vi "example.vi"() -> ()   [LabVIEW 2015]
uses:
  SubVI/lstsqr_lines.vi
  SubVI/z-split sum difference.vi
  SubVI/Local gradient preallocation.vi
  <vilib>/vision/NI_Vision_Development_Module.lvlib
panel:
  in  "Image type":u16(ring) items=["Fluorescent", "Brightfield"]
  in  "pattern":string="*.*"
  in  "Current im":u16=5 caption="Current image" max=0 step=1
  out "ImageArray":u16[][][](array[numeric])
  in  "Express btn":bool
  in  "Positive angle":dbl
  out "Show center":bool
  out "Z plot":cluster{i32[], "XYZ":dbl[]}(graph)
  out "Y plot":cluster{i32[], "XYZ":dbl[]}(graph)
  out "X plot":cluster{i32[], "XYZ":dbl[]}(graph)
  out "Gx graph":dbl[][](graph)
  in  "Center size":dbl=5.0 min=1.0 step=2.0
  out "Center":dbl[](array[numeric]) format="%#.5g"
  out "Weights":dbl[](array[numeric])
  out "gradients":dbl[][](array[numeric])
  out "centers":i32[][](array[numeric])
  in  "Gradient btn":bool
  out "Gy graph":dbl[][](graph)
  out "G graph":dbl[][](graph)
  in  "Threshold type":u16(ring) items=["Top fraction", "Top value"]
  in  "Weights type":u16(ring)=1 items=["None", "G", "G^2"]
  in  "Threshold":dbl=2.0
  in  "R":dbl=10.0
  in  "Center Button":bool
  in  "Stop Button":bool
  in  "Read Button":bool
  out "Input image":T1(plugin-control)
  in  "File Path":path
  out "Filtered G":dbl[][](graph)
  # "Run vi. \n1. Use default image or select a greyscale image and click Read. There is an option to select either directory or a file. If directory is selected, Labview will read all the files in the folder AND in ALL subfolders. You can use a \"pattern\" field to select specific files.\n2. Select an image type: Fluorescent or Brightfield (affect z-calculation)\n3. Set parameters R, Threshold, Weights type, Positive angle, etc.\n4. A. Single file\n    OPTION1. Step by step: \n      - click Gradient to calculate local gradient images\n      - click Find center to calculate xyz position of the particle\n    OPTION2. Express: \n      - click Express center\n\n   B. Folder\n    OPTION1. Step by step: \n      - click Gradient to calculate local gradient images for the image selected in Current image\n      - click Find center to calculate xyz position of the particle for the image selected in Current image\n    OPTION2. Express: \n      - click Express center to find center for all the loaded files\n\nAuthor: Anatolii Kashchuk"
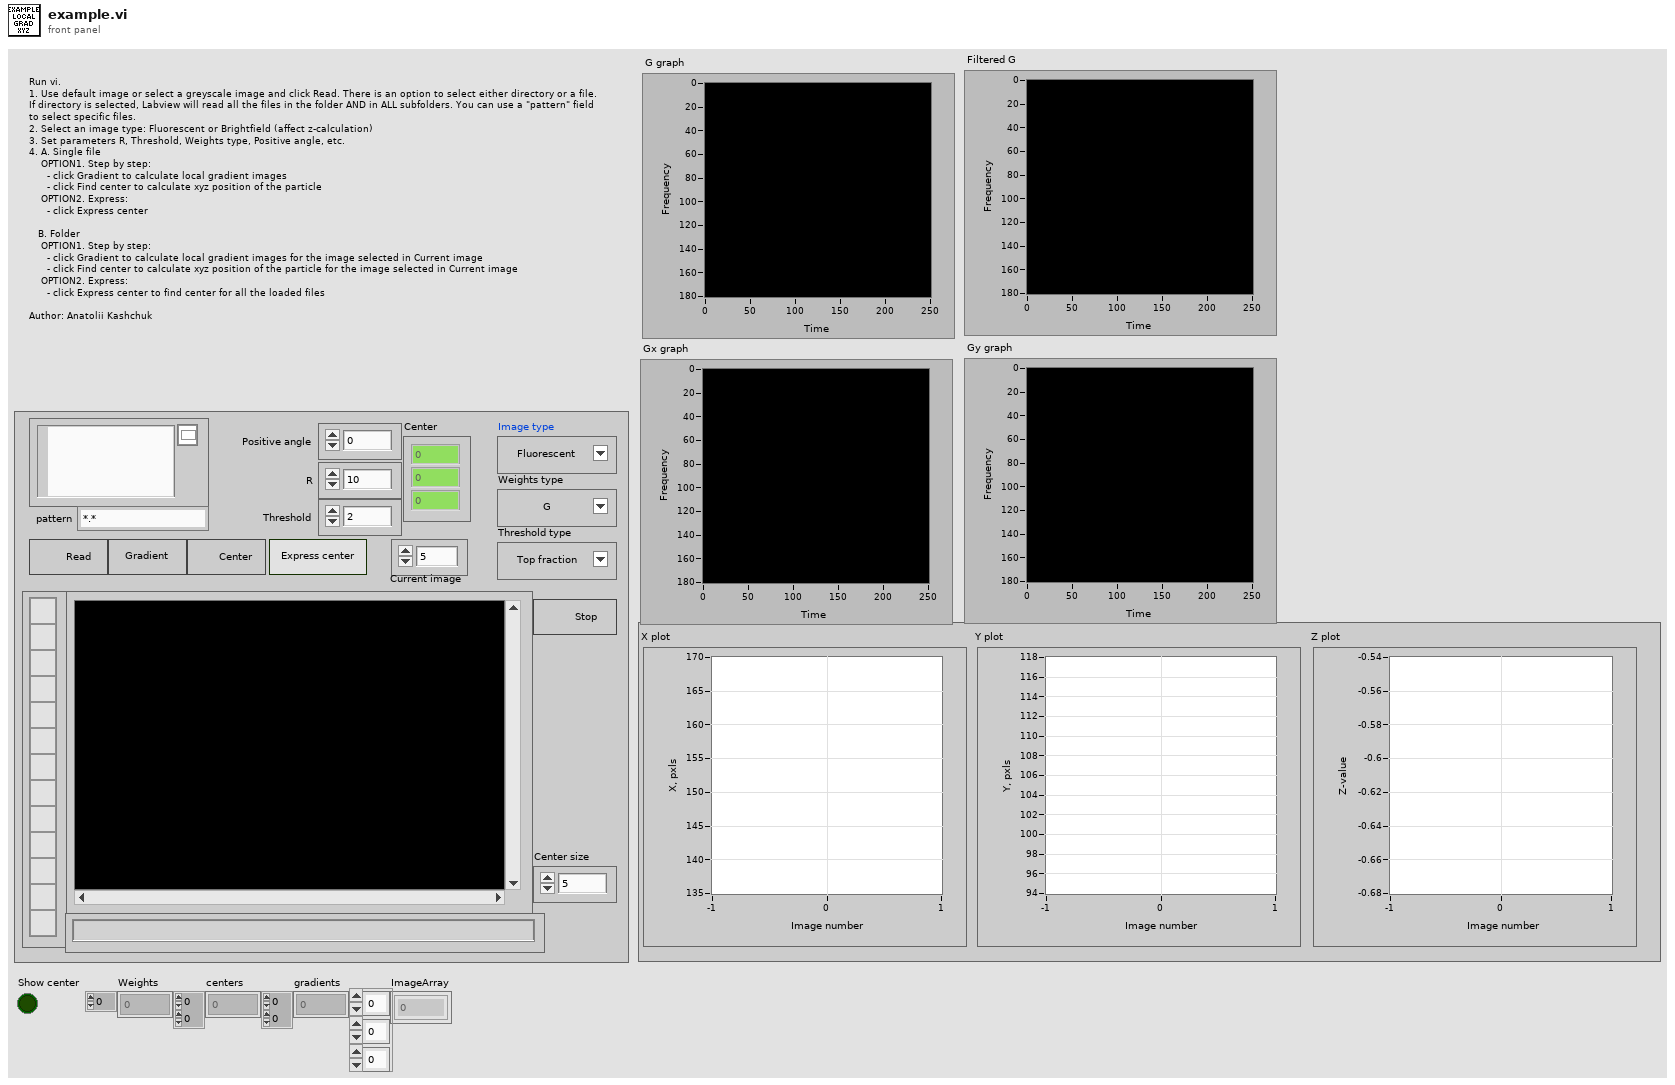
[diagram p1: front panel]
types:
  T1 = typedef "IMAQ Image.ctl" = refnum<image>
  T2 = typedef "Image Type" = u32
  T3 = cluster{"Left":i32, "Top":i32, "Right":i32, "Bottom":i32}
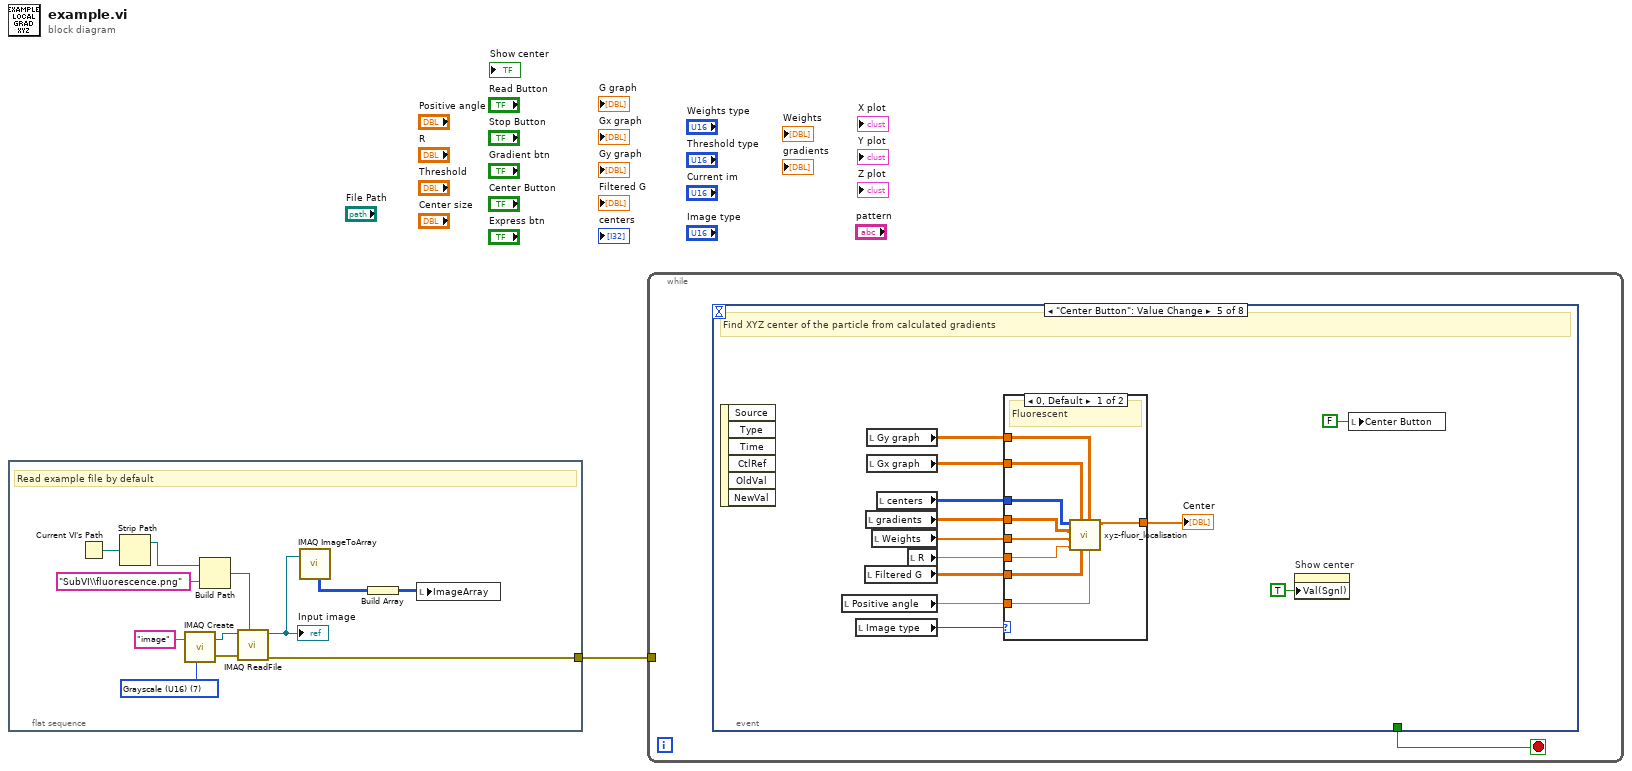
[diagram p0: block diagram]
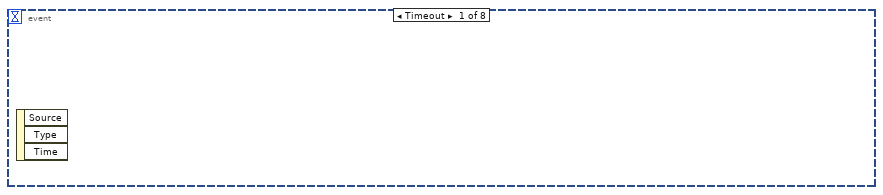
[diagram p2: hidden frame]
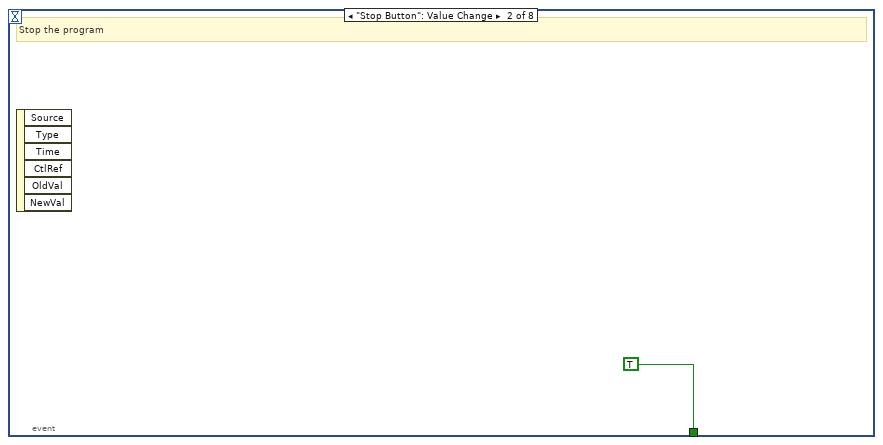
[diagram p3: hidden frame]
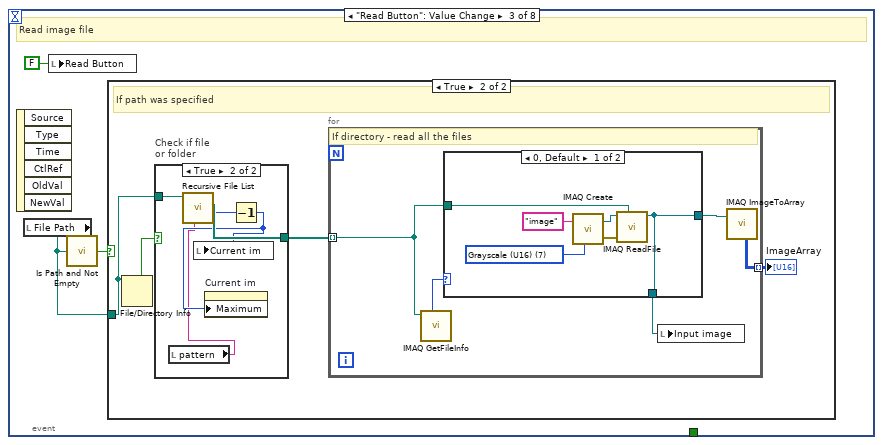
[diagram p4: hidden frame]
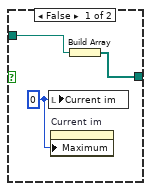
[diagram p6: hidden frame]
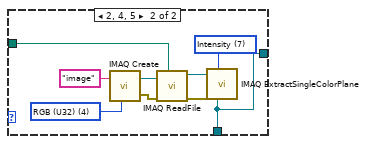
[diagram p7: hidden frame]
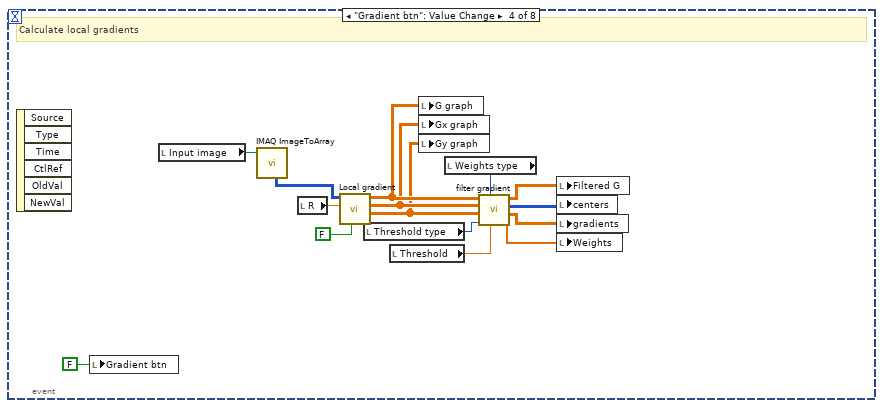
[diagram p8: hidden frame]
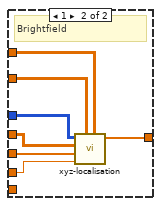
[diagram p9: hidden frame]
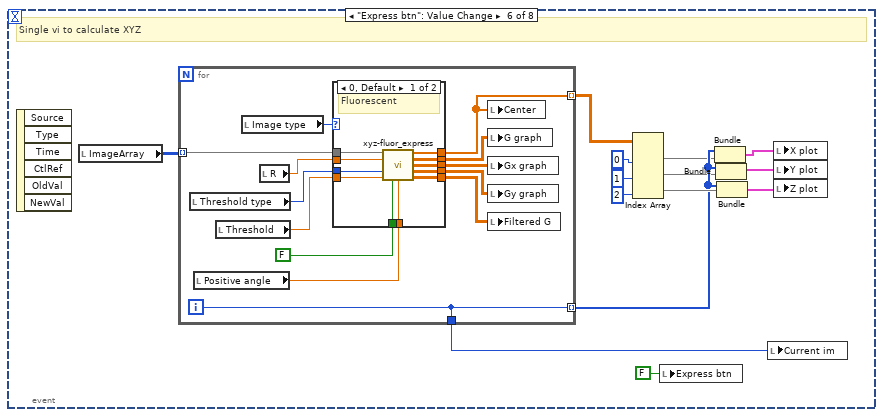
[diagram p10: hidden frame]
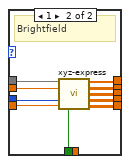
[diagram p11: hidden frame]
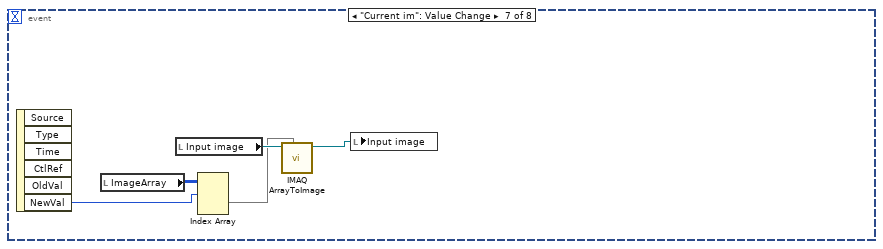
[diagram p12: hidden frame]
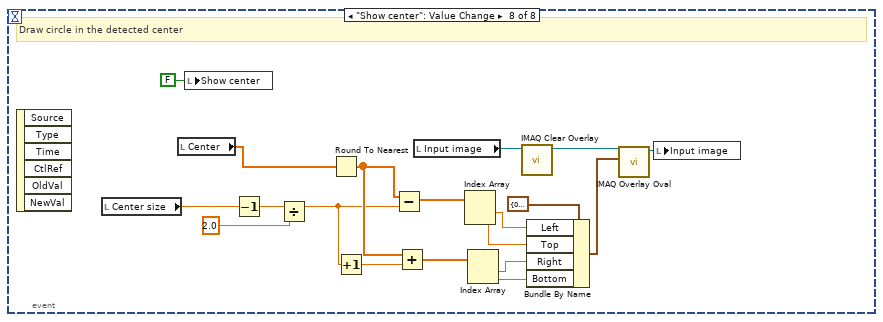
[diagram p13: hidden frame]
diagram:
  n1 = flat-sequence {
    tunnel: [w10] -> w1
    frame #0 {
      w9 = T2 7 items=["Grayscale (U8)", "Grayscale (I16)", "Grayscale (SGL)", "Complex (CSG)", "RGB (U32)", "HSL (U32)", "RGB (U64)", "Grayscale (U16)"] ("Image Type")
      # "Read example file by default"
      n2 = Current VI's Path() -> (path=w7:path)
      n3 = Strip Path(path=w7) -> (stripped path=w5:path)  [unwired: 1 out]
      n4 = call "IMAQ Create"("Image Name"="image", "Image Type"=w9) -> ("New Image"=w11:T1, "error out"=w12:errorcluster)  [unwired: 3 in]
      n5 = Build Path(base path=w5, name or relative path="SubVI\\fluorescence.png") -> (appended path=w6:path)
      n6 = call "IMAQ ReadFile"("File Path"=w6, "error in (no error)"=w12, "Image"=w11) -> ("error out"=w10:errorcluster, "Image Out"=w4:T1)  [unwired: 4 in, 3 out]
      "Input image" <- w4
      n7 = call "IMAQ ImageToArray"("Image"=w4) -> ("Image Pixels (U16)"=w2:u16[][])  [unwired: 3 in, 4 out]
      n8 = Build Array(w2) -> (w3:u16[][][])
      n9 = local write "ImageArray"(w3) -> ()
    }
  }
  n10 = while {
    tunnel: w1 -> [_]
    stop <- w14 stop-if-true
    n11 = event shown="[4] \"Center Button\": Value Change" {
      selector: _ -> [_ _ _ _ _ _ _ _]
      dyn-events: _ -> [_ _ _ _ _ _ _ _]
      timeout: _ -> [_ _ _ _ _ _ _ _]
      tunnel: [_ TRUE _ _ _ _ _ _] -> w14
      event Timeout {
        n12 = event-data() -> ()  [unwired: 1 in, 3 out]
      }
      event "Stop Button": Value Change {
        # "Stop the program"
        n13 = event-data() -> ()  [unwired: 1 in, 6 out]
      }
      event "Read Button": Value Change {
        # "Read image file"
        n14 = event-data() -> ()  [unwired: 1 in, 6 out]
        n15 = local read "File Path"() -> (w17:path)
        n16 = local write "Read Button"(FALSE ("Read Button")) -> ()
        n17 = call <vilib>:"Is Path and Not Empty.vi"("path"=w17) -> ("Is Path and Not Empty?"=w16:bool)  [unwired: 4 in]
        n18 = case shown="True" w16 {
          tunnel: w17 -> [_ w22]
          frame False {
          }
          frame True {
            # "If path was specified"
            n19 = File/Directory Info(path=w22) -> (directory=w21:bool)  [unwired: 1 in, 6 out]
            n20 = case "Check if file \nor folder" shown="True" w21 {
              tunnel: w22 -> [w25 w30]
              tunnel: [w24 w29] -> w20
              frame False {
                w23 = u16 0 ("Current im")
                n21 = local write "Current im"(w23) -> ()
                n22 = property on="Current im" class="DigNum (strict)"("Maximum"=w23) -> ()  [unwired: 2 in, 2 out]
                n23 = Build Array(w25) -> (w24:path[])
              }
              frame True {
                n24 = local read "pattern"() -> (w26:string)
                n25 = call <vilib>:"Recursive File List.vi"("pattern"=w26, "Folder Path"=w30) -> ("Number of Files"=w28:i32, "All Files in Dir"=w29:path[])  [unwired: 5 in, 3 out]
                n26 = Decrement(x=w28) -> (x-1=w27:i32)
                n27 = local write "Current im"(w27) -> ()
                n28 = property on="Current im" class="DigNum (strict)"("Maximum"=w27) -> ()  [unwired: 2 in, 2 out]
              }
            }
            n29 = for {
              tunnel: w20 -> [w35] mode=indexing
              tunnel: [w31] -> w19 mode=indexing
              # "If directory - read all the files"
              n30 = call "IMAQ GetFileInfo"("File Path"=w35) -> ("Image Type"=w34:T2)  [unwired: 4 in, 6 out]
              n31 = case shown="0, Default" w34 {
                tunnel: [w36 w42] -> w33
                tunnel: w35 -> [w37 w44]
                tunnel: [w36 w42] -> w32
                frame 0, Default {
                  w41 = T2 7 items=["Grayscale (U8)", "Grayscale (I16)", "Grayscale (SGL)", "Complex (CSG)", "RGB (U32)", "HSL (U32)", "RGB (U64)", "Grayscale (U16)"] ("Image Type")
                  n32 = call "IMAQ Create"("Image Name"="image", "Image Type"=w41) -> ("New Image"=w39:T1, "error out"=w38:errorcluster)  [unwired: 3 in]
                  n33 = call "IMAQ ReadFile"("File Path"=w37, "error in (no error)"=w38, "Image"=w39) -> ("Image Out"=w36:T1)  [unwired: 4 in, 4 out]
                }
                frame 2, 4, 5 {
                  w46 = T2 4 items=["Grayscale (U8)", "Grayscale (I16)", "Grayscale (SGL)", "Complex (CSG)", "RGB (U32)", "HSL (U32)", "RGB (U64)", "Grayscale (U16)"] ("Image Type")
                  w50 = 7 items=["Red", "Green", "Blue", "Hue", "Saturation", "Luminance", "Value", "Intensity"] ("Color Plane")
                  n34 = call "IMAQ Create"("Image Name"="image", "Image Type"=w46) -> ("New Image"=w45:T1, "error out"=w43:errorcluster)  [unwired: 3 in]
                  n35 = call "IMAQ ReadFile"("File Path"=w44, "error in (no error)"=w43, "Image"=w45) -> ("error out"=w48:errorcluster, "Image Out"=w49:T1)  [unwired: 4 in, 3 out]
                  n36 = call "IMAQ ExtractSingleColorPlane"("Color Plane"=w50, "error in (no error)"=w48, "Image Src"=w49) -> ("Image Dst Out"=w42:T1)  [unwired: 7 in, 1 out]
                }
              }
              n37 = local write "Input image"(w33) -> ()
              n38 = call "IMAQ ImageToArray"("Image"=w32) -> ("Image Pixels (U16)"=w31:u16[][])  [unwired: 3 in, 4 out]
            }
            "ImageArray" <- w19
          }
        }
      }
      event "Gradient btn": Value Change {
        # "Calculate local gradients"
        n39 = event-data() -> ()  [unwired: 1 in, 6 out]
        n40 = local write "Gradient btn"(FALSE ("Center Button")) -> ()
        n41 = local read "Input image"() -> (w64:T1)
        n42 = call "IMAQ ImageToArray"("Image"=w64) -> ("Image Pixels (U16)"=w62:u16[][])  [unwired: 3 in, 4 out]
        n43 = local read "R"() -> (w63:dbl)
        n44 = call "Local gradient.vi"("FFT allocated?"=FALSE, "R"=w63, "Image"=w62) -> ("Gy"=w59:dbl[][], "Gx"=w60:dbl[][], "G"=w61:dbl[][])  [unwired: 6 in]
        n45 = local read "Threshold type"() -> (w52:u16)
        n46 = local read "Threshold"() -> (w53:dbl)
        n47 = local write "G graph"(w61) -> ()
        n48 = local write "Gx graph"(w60) -> ()
        n49 = local write "Gy graph"(w59) -> ()
        n50 = local read "Weights type"() -> (w54:u16)
        n51 = call "filter gradient.vi"("Threshold"=w53, "Weights type"=w54, "Threshold type"=w52, "Gy"=w59, "Gx"=w60, "G"=w61) -> ("Weights"=w56:dbl[], "gradients"=w55:dbl[][], "centers"=w57:i32[][], "Filtered G"=w58:dbl[][])  [unwired: 2 out]
        n52 = local write "Filtered G"(w58) -> ()
        n53 = local write "centers"(w57) -> ()
        n54 = local write "gradients"(w55) -> ()
        n55 = local write "Weights"(w56) -> ()
      }
      event "Center Button": Value Change {
        # "Find XYZ center of the particle from calculated gradients"
        n56 = event-data() -> ()  [unwired: 1 in, 6 out]
        n57 = local read "Positive angle"() -> (w67:dbl)
        n58 = local read "Image type"() -> (w66:u16)
        n59 = local read "Filtered G"() -> (w68:dbl[][])
        n60 = local read "gradients"() -> (w74:dbl[][])
        n61 = local read "Gy graph"() -> (w70:dbl[][])
        n62 = local read "Gx graph"() -> (w69:dbl[][])
        n63 = local read "Weights"() -> (w73:dbl[])
        n64 = local read "centers"() -> (w75:i32[][])
        n65 = local read "R"() -> (w72:dbl)
        n66 = case shown="0, Default" w66 {
          tunnel: w75 -> [w86 w90]
          tunnel: w74 -> [w85 w89]
          tunnel: w73 -> [w84 w88]
          tunnel: w72 -> [w83 w87]
          tunnel: [w82 w93] -> w71
          tunnel: w70 -> [w81 w92]
          tunnel: w69 -> [w80 w91]
          tunnel: w68 -> [w79 _]
          tunnel: w67 -> [w78 _]
          frame 0, Default {
            # "Fluorescent"
            n67 = call "xyz-fluor_localisation.vi"("Positive angle"=w78, "Gy"=w81, "Gthr"=w79, "Gx"=w80, "R"=w83, "weights"=w84, "B points"=w85, "A points"=w86) -> ("XYZ"=w82:dbl[])  [unwired: 2 in, 1 out]
          }
          frame 1 {
            # "Brightfield"
            n68 = call "xyz-localisation.vi"("Gy"=w92, "Gx"=w91, "R"=w87, "weights"=w88, "B points"=w89, "A points"=w90) -> ("XYZ"=w93:dbl[])  [unwired: 4 in, 1 out]
          }
        }
        "Center" <- w71
        n69 = property on="Show center" class="Bool (strict)"("Val(Sgnl)"=TRUE ("Value (Signaling)")) -> ()  [unwired: 2 in, 2 out]
        n70 = local write "Center Button"(FALSE ("Center Button")) -> ()
      }
      event "Express btn": Value Change {
        # "Single vi to calculate XYZ"
        n71 = event-data() -> ()  [unwired: 1 in, 6 out]
        n72 = local read "ImageArray"() -> (w106:u16[][][])
        n73 = for {
          tunnel: w106 -> [w110] mode=indexing
          tunnel: [w111] -> w105 mode=indexing
          tunnel: [w109] -> w100 mode=indexing
          tunnel: [w109] -> w94
          i -> [w109]
          n74 = local read "Threshold type"() -> (w119:u16)
          n75 = local read "Positive angle"() -> (w117:dbl)
          n76 = local read "Threshold"() -> (w118:dbl)
          n77 = local read "Image type"() -> (w108:u16)
          n78 = local read "R"() -> (w120:dbl)
          n79 = case shown="0, Default" w108 {
            tunnel: w120 -> [w131 w135]
            tunnel: w119 -> [w130 w134]
            tunnel: w118 -> [w129 w133]
            tunnel: w117 -> [w128 _]
            tunnel: FALSE ("FFT allocated?") -> [w127 w132]
            tunnel: [w126 w140] -> w115
            tunnel: [w125 w139] -> w114
            tunnel: [w124 w138] -> w113
            tunnel: [w123 w137] -> w112
            tunnel: [w122 w141] -> w111
            tunnel: w110 -> [w121 w136]
            frame 0, Default {
              # "Fluorescent"
              n80 = call "xyz-fluor_express.vi"("Image"=w121, "R"=w131, "Threshold type"=w130, "Threshold"=w129, "FFT allocated?"=w127, "Positive angle"=w128) -> ("XYZ"=w122:dbl[], "G"=w126:dbl[][], "Gx"=w125:dbl[][], "Gy"=w124:dbl[][], "Filtered G"=w123:dbl[][])  [unwired: 4 in, 1 out]
            }
            frame 1 {
              # "Brightfield"
              n81 = call "xyz-express.vi"("Image"=w136, "R"=w135, "Threshold type"=w134, "Threshold"=w133, "FFT allocated?"=w132) -> ("XYZ"=w141:dbl[], "G"=w140:dbl[][], "Gx"=w139:dbl[][], "Gy"=w138:dbl[][], "Filtered G"=w137:dbl[][])  [unwired: 5 in, 1 out]
            }
          }
          n82 = local write "Center"(w111) -> ()
          n83 = local write "G graph"(w115) -> ()
          n84 = local write "Gx graph"(w114) -> ()
          n85 = local write "Gy graph"(w113) -> ()
          n86 = local write "Filtered G"(w112) -> ()
        }
        n87 = Index Array(array=w105, index (col) #1=0 ("disabled index (col)"), index (col) #2=1 ("index (col)"), index (col) #3=2 ("index (col)")) -> (element #1=w99:dbl[], element #2=w98:dbl[], element #3=w101:dbl[])  [unwired: 3 in]
        n88 = local write "Express btn"(FALSE ("Express btn")) -> ()
        n89 = Bundle(w100, "XYZ"=w99) -> (w97:cluster{i32[], "XYZ":dbl[]})  [unwired: 1 in]
        n90 = Bundle(w100, "XYZ"=w98) -> (w96:cluster{i32[], "XYZ":dbl[]})  [unwired: 1 in]
        n91 = Bundle(w100, "XYZ"=w101) -> (w95:cluster{i32[], "XYZ":dbl[]})  [unwired: 1 in]
        n92 = local write "Current im"(w94) -> ()
        n93 = local write "X plot"(w97) -> ()
        n94 = local write "Y plot"(w96) -> ()
        n95 = local write "Z plot"(w95) -> ()
      }
      event "Current im": Value Change {
        n96 = event-data() -> ("NewVal"=w143:u16)  [unwired: 1 in, 5 out]
        n97 = local read "ImageArray"() -> (w144:u16[][][])
        n98 = local read "Input image"() -> (w146:T1)
        n99 = Index Array(array=w144, index (dim 0)=w143) -> (element=w142:u16[][])  [unwired: 2 in]
        n100 = call "IMAQ ArrayToImage"("Image Pixels (U16)"=w142, "Image"=w146) -> ("Image Out"=w145:T1)  [unwired: 8 in, 1 out]
        n101 = local write "Input image"(w145) -> ()
      }
      event "Show center": Value Change {
        # "Draw circle in the detected center"
        n102 = event-data() -> ()  [unwired: 1 in, 6 out]
        n103 = local read "Center size"() -> (w163:dbl)
        n104 = local read "Center"() -> (w148:dbl[])
        n105 = local write "Show center"(FALSE ("Show center")) -> ()
        n106 = Decrement(x=w163) -> (x-1=w153:dbl)
        n107 = Divide(x=w153, y=2.0) -> (x/y=w152:dbl)
        n108 = Round To Nearest(number=w148) -> (nearest integer value=w155:dbl[])
        n109 = Increment(x=w152) -> (x+1=w151:dbl)
        n110 = Subtract(x=w155, y=w152) -> (x-y=w164:dbl[])
        n111 = Add(x=w155, y=w151) -> (x+y=w160:dbl[])
        n112 = local read "Input image"() -> (w150:T1)
        n113 = Index Array(array=w164) -> (element #1=w162:dbl, element #2=w161:dbl)  [unwired: 2 in]
        n114 = Index Array(array=w160) -> (element #1=w159:dbl, element #2=w158:dbl)  [unwired: 2 in]
        n115 = call "IMAQ Clear Overlay"("Image"=w150) -> ("Image Out"=w149:T1)  [unwired: 9 in, 1 out]
        n116 = Bundle By Name(cluster=T3 {"Left"=0, "Top"=0, "Right"=0, "Bottom"=0} ("Bounding Rectangle"), "Left"=w162, "Top"=w161, "Right"=w159, "Bottom"=w158) -> (w156:T3)
        n117 = call "IMAQ Overlay Oval"("Bounding Rectangle"=w156, "Image"=w149) -> ("Image Out"=w157:T1)  [unwired: 8 in, 1 out]
        n118 = local write "Input image"(w157) -> ()
      }
    }
  }
